vi "Pigeon.vi"(10 "Can ID":u8) -> ()   [LabVIEW 2019]
uses:
  <vilib>/Rock Robotics/WPI/ThirdParty/Phoenix-LabVIEW/Pigeon IMU/CTRE_PigeonIMU_TareType.ctl
  <vilib>/Rock Robotics/WPI/ThirdParty/Phoenix-LabVIEW/Pigeon IMU/CTRE_PigeonIMU_Open_TalonSRX.vi
  <vilib>/Rock Robotics/WPI/ThirdParty/Phoenix-LabVIEW/Pigeon IMU/CTRE_PigeonIMU_GetYPR.vi
  Drive Global.vi
panel:
  out "Yaw Pitch Roll":cluster{"Yaw":dbl, "Pitch":dbl, "Roll":dbl}
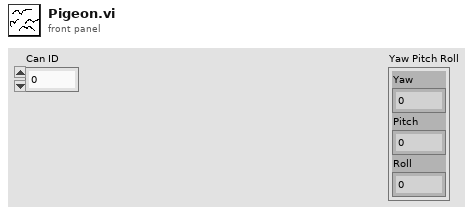
[diagram p1: front panel]
types:
  T1 = typedef "WPI_MotorControlDeviceRef.ctl" = cluster{"DeviceStatus":errorcluster, "Type":T2, "PWM":cluster{"PWM Channel":T3, "DeadBand":T4}, "CAN":cluster{"Device Number":u8, "SetOutput VI Ref":variant, "GetOutput VI Ref":variant, "Enable VI Ref":variant, "Disable VI Ref":variant, "Data":variant}, "Invert":bool, "DIO PWM":cluster{"PWM \"Enable\" Channel":T3, "DIOChannel":T5, "PWM Rate":dbl}}
  T2 = typedef "WPI_MotorControlType.ctl" = enum16{"PWM", "CAN", "DIO PWM"}
  T3 = typedef "FPGA_DIOPWMChannel.ctl" = enum8{"PWM 0", "PWM 1", "PWM 2", "PWM 3", "PWM 4", "PWM 5", "PWM 6", "PWM 7", "PWM 8", "PWM 9", "PWM MXP 0", "PWM MXP 1", "PWM MXP 2", "PWM MXP 3", "PWM MXP 4", "PWM MXP 5", "PWM MXP 6", "PWM MXP 7", "PWM MXP 8", "PWM MXP 9", "Invalid"}
  T4 = typedef "WPI_PWMDeadband.ctl" = cluster{"Name":string, "maxPositivePwm":i32, "minPositivePwm":i32, "centerPwm":i32, "maxNegativePwm":i32, "minNegativePwm":i32, "angularRange":u16}
  T5 = typedef "FPGA_DIOChannel.ctl" = enum8{"DIO 0", "DIO 1", "DIO 2", "DIO 3", "DIO 4", "DIO 5", "DIO 6", "DIO 7", "DIO 8", "DIO 9", "DIO MXP 0", "DIO MXP 1", "DIO MXP 2", "DIO MXP 3", "DIO MXP 4", "DIO MXP 5", "DIO MXP 6", "DIO MXP 7", "DIO MXP 8", "DIO MXP 9", "DIO MXP 10", "DIO MXP 11", "DIO MXP 12", "DIO MXP 13", "DIO MXP 14", "DIO MXP 15", "SPI Port CS1", "SPI Port CS2", "SPI Port CS3", "SPI Port MISO", "SPI Port MOSI", "Invalid"}
  T6 = typedef "CTRE_PigeonIMU_DeviceRef.ctl" = cluster{"DeviceStatus":errorcluster, "Device Number":u8, "Type":T7, "Device ID":u32, "Handle":u64, "UsageFrame":u32, "Library Path":path}
  T7 = typedef "CTRE_PigeonIMU_ConnectionType.ctl" = u32
  T8 = typedef "CTRE_PigeonIMU_TareType.ctl" = u8
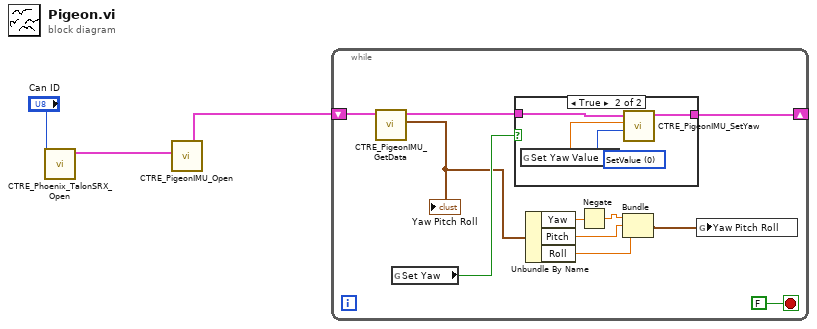
[diagram p0: block diagram]
diagram:
  n1 = call <vilib>:"CTRE_Phoenix_TalonSRX_Open.vi"("Device Number"="Can ID") -> ("CAN Talon SRX Ref"=w3:T1)  [unwired: 9 in, 1 out]
  n2 = call-poly <vilib>:"CTRE_PigeonIMU_Open.vi"("CAN Talon SRX Ref"=w3) -> ("PigeonIMUDevRef"=w2:T6)  [unwired: 9 in, 1 out]
  n3 = while {
    shift-right: [w11] -> _
    shift-left: w2 -> [w13]
    stop <- FALSE stop-if-true
    n4 = call-poly <vilib>:"CTRE_PigeonIMU_GetData.vi"("PigeonIMUDevRef"=w13) -> ("Yaw Pitch Roll"=w9:cluster{"Yaw":dbl, "Pitch":dbl, "Roll":dbl}, "PigeonIMUDevRef"=w12:T6)  [unwired: 8 in, 1 out]
    "Yaw Pitch Roll" <- w9
    n5 = global read "Drive Global.vi" "Set Yaw"() -> (w10:bool)
    n6 = case shown="True" w10 {
      tunnel: w12 -> [w15 w18]
      tunnel: [w15 w17] -> w11
      frame False {
      }
      frame True {
        w19 = T8 0 items=["SetValue"=0, "AddOffset"=1, "MatchCompass"=2, "SetOffset"=255] ("TareType (SetValue)")
        n7 = global read "Drive Global.vi" "Set Yaw Value"() -> (w16:dbl)
        n8 = call <vilib>:"CTRE_PigeonIMU_SetYaw.vi"("TareType (SetValue)"=w19, "Value"=w16, "PigeonIMUDevRef"=w18) -> ("PigeonIMUDevRef"=w17:T6)  [unwired: 7 in, 1 out]
      }
    }
    n9 = Unbundle By Name(w9) -> ("Yaw"=w8:dbl, "Pitch"=w6:dbl, "Roll"=w5:dbl)
    n10 = Negate(x=w8) -> (-x=w7:dbl)
    n11 = Bundle(w7, "Pitch"=w6, "Roll"=w5) -> (w4:cluster{dbl, "Pitch":dbl, "Roll":dbl})  [unwired: 1 in]
    n12 = global write "Drive Global.vi" "Yaw Pitch Roll"(w4) -> ()
  }
